vi "SPC_stop_measurement.vi"(8 "Error In":errorcluster, 10 "Module No":i16 min=0 max=7 step=1, 11 "DLL Path":path) -> (0 "Error Out":errorcluster, 2 "Module No":i16, 3 "DLL Path":path)   [LabVIEW 2023]
doc: "The procedure is used to terminate a running measurement on the SPC module ‘mod_no’. \nBecause of hardware differences the procedure's action varies for different SPC module types.\nFor all SPC module types (except SPC-6x0/13x/830/140/930/15x/160 in FIFO mode):\nIf the sequencer is not enabled (normal measurement):\n - The SPC is disarmed (i.e. the photon collection is stopped)\n - The repeat and collection timers are read to get the break times\nWhen the sequencer is enabled:\n - The sequencer is stopped\n - The SPC is disarmed (photon collection is stopped)\nThe procedure should be called after finished scan mode measurement to stop the sequencer and clear scan flags (SPC_FBRDY).\nFor all SPC module types (except SPC-6x0/130/131) in SCAN_IN mode:\nIf the measurement was started in SCAN_IN mode, 1st call to the function forces very short collection time to finish the current frame and returns error -21. The measurement will stop automatically after finishing current frame. 2nd call will stop the measurement without waiting for the end of frame.\nFor SPC-6x0/13x/830/140/930/15x/160 in FIFO mode:\n- The SPC is disarmed (photon collection is stopped)\n- The FIFO pipeline is cleared\nFor SPC-830/140/15x/160 in FIFO_32M mode ( Fifo Image ):\nThe functionality is added which enables higher level software to stop the measurement after collecting the whole frames.\nStopping the measurement requires two calls of SPC_stop_measurement.\n1st call of SPC_stop_measurement:\n- photon collection is not yet stopped\n- current position of write pointer of FIFO is remembered as a stop position -\nsubsequent SPC_read_fifo calls will return 1 when this place in FIFO is reached - this is a sign for higher level software that all photons collected up to the stop moment were read. From this moment photons should be read until a frame marker will appear in photons stream - then higher level software should call SPC_stop_measurement again to stop collecting photons. \n2nd call of SPC_stop_measurement:\n- The SPC is disarmed (photon collection is stopped)\n- The FIFO pipeline is cleared\n\ninfo@becker-hickl.com"
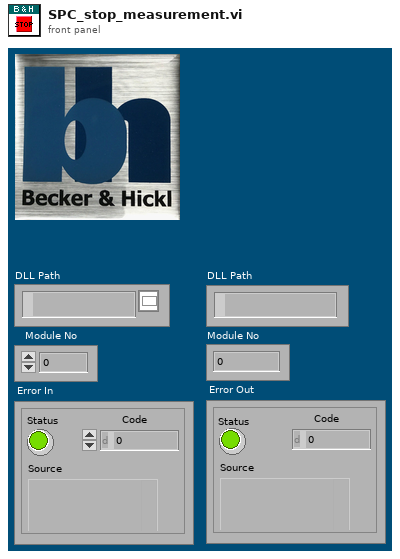
[diagram p1: front panel]
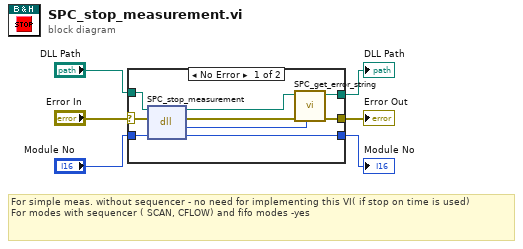
[diagram p0: block diagram]
diagram:
  # "For simple meas. without sequencer - no need for implementing this VI( if stop on time is used)\nFor modes with sequencer ( SCAN, CFLOW) and fifo modes -yes"
  n1 = case shown="No Error" "Error In" {
    selector: "Error In" -> [w15 w17]
    tunnel: [w7 w17] -> w5
    tunnel: "DLL Path" -> [w14 w18]
    tunnel: [w10 w18] -> w3
    tunnel: [w12 w16] -> w2
    tunnel: "Module No" -> [w11 w16]
    frame No Error {
      n2 = dll-call lib="D:/spcm/lib/lab_view/lv10.0/spcm32.dll" fn="SPC_stop_measurement"(path in=w14, error in=w15, "mod_no"=w11) -> (path out=w13:path, error out=w8:errorcluster, "return type"=w9:i16, "mod_no"=w12:i16)  [unwired: 1 in]
      n3 = call "SPC_get_error_string.vi"("ErrorID"=w9, "Error In"=w8, "DLL Path"=w13) -> ("Error Out"=w7:errorcluster, "DLL Path"=w10:path)  [unwired: 6 in, 1 out]
    }
    frame Error {
    }
  }
  "Error Out" <- w5
  "DLL Path" <- w3
  "Module No" <- w2
